vi "CheckIfViIsLoadedInSubPanel.vi"(8 "error in (no error)":errorcluster, 11 "vi reference":refnum<vi>) -> (0 "error out":errorcluster, 1 "In SubPanel?":bool, 3 "VI reference out":refnum<vi>)   [LabVIEW 2018, in "Visualization.lvlib" / "VisualizeBase.lvclass"]
uses:
  VisualizeBase.lvclass
  SubVI/VisualizationManagement/VisualizationManagerActions.ctl
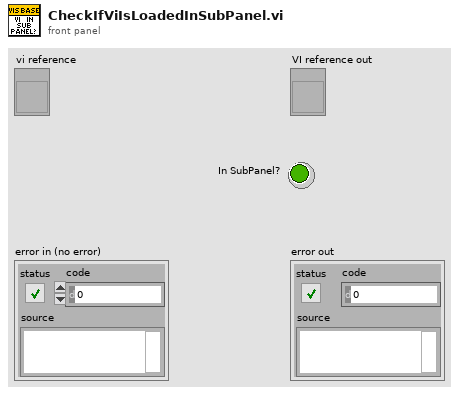
[diagram p1: front panel]
types:
  T1 = typedef "VisualizationManagerActions.ctl" = enum16{"Set", "LoadModVI", "PopInOutModVI", "Add", "Clear", "CloseVisMod", "LoadLatestModule", "Get"}
  T2 = enum32{"Invalid", "Standard", "Closed", "Hidden", "Minimized", "Maximized"}
  T3 = typedef "OpenVisualizationVIs.ctl" = cluster{"Module Name":string, "VI ref":refnum<vi>, "In SubPanel?":bool, "Time Stamp":timestamp}
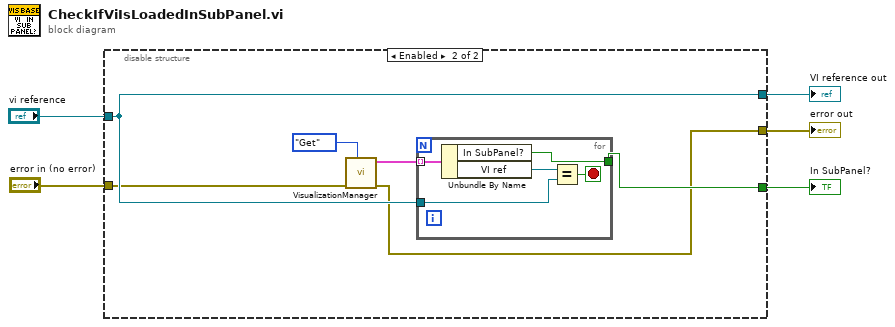
[diagram p0: block diagram]
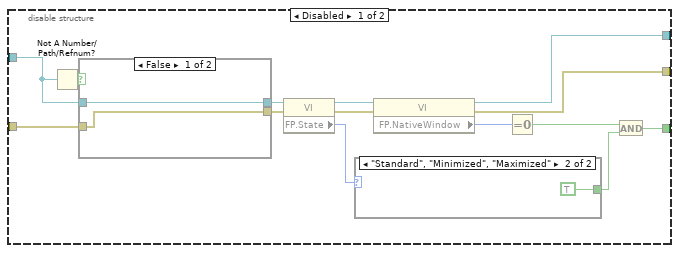
[diagram p2: hidden frame]
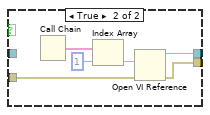
[diagram p3: hidden frame]
diagram:
  n1 = disable-structure shown="Enabled" {
    disable-tunnel: [w13 w31] -> w5
    disable-tunnel: [w10 w29] -> w4
    disable-tunnel: "error in (no error)" -> [w9 w30]
    disable-tunnel: "vi reference" -> [w7 w32]
    disable-tunnel: [w6 w32] -> w1
    frame Disabled {
      n2 = Not A Number/Path/Refnum?(number/path/refnum=w7) -> (NaN/Path/Refnum?=w8:bool)
      n3 = case shown="False" w8 {
        tunnel: [w21 w24] -> w12
        tunnel: [w20 w23] -> w11
        tunnel: w9 -> [w20 w22]
        tunnel: w7 -> [w21 _]
        frame False {
        }
        frame True {
          n4 = Call Chain() -> (call chain=w27:string[])
          n5 = Index Array(array=w27, index=1) -> (element=w25:string)
          n6 = Open VI Reference(vi path=w25, error in (no error)=w22) -> (vi reference=w24:refnum<vi>, error out=w23:errorcluster)  [unwired: 4 in]
        }
      }
      n7 = property class="VI"(reference=w12, error in=w11) -> (reference out=w17:refnum<vi>, error out=w18:errorcluster, "FP.State"=w19:T2)
      n8 = case shown="\"Standard\", \"Minimized\", \"Maximized\"" w19 {
        tunnel: [_ TRUE] -> w15
        frame Default {
        }
        frame "Standard", "Minimized", "Maximized" {
        }
      }
      n9 = property class="VI"(reference=w17, error in=w18) -> (reference out=w6:refnum<vi>, error out=w10:errorcluster, "FP.NativeWindow"=w16:u64)
      n10 = Equal To 0?(x=w16) -> (x = 0?=w14:bool)
      n11 = And(x=w14, y=w15) -> (x .and. y?=w13:bool)
    }
    frame Enabled {
      n12 = call "VisualizationManager.vi"("Action"=VisualizationManagerActions."Get", "error in (no error)"=w30) -> ("error out"=w29:errorcluster, "Open Visualization VIs out"=w33:T3[])  [unwired: 6 in, 2 out]
      n13 = for {
        tunnel: w33 -> [w39] mode=indexing
        tunnel: w32 -> [w37]
        tunnel: [w35] -> w31
        stop <- w36 stop-if-true
        n14 = Unbundle By Name(w39) -> ("In SubPanel?"=w35:bool, "VI ref"=w38:refnum<vi>)
        n15 = Equal?(x=w38, y=w37) -> (x = y?=w36:bool)
      }
    }
  }
  "In SubPanel?" <- w5
  "error out" <- w4
  "VI reference out" <- w1
